vi "User events.vi"() -> (0 "error out":errorcluster, 3 "User events":T1)   [LabVIEW 2020, in "Arduino stepper.lvlib"]
uses:
  Arduino stepper.lvlib
  Wake HL args--typedef.ctl
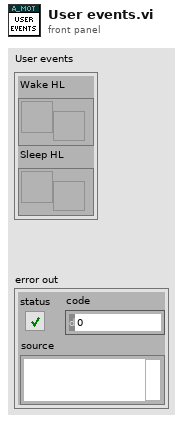
[diagram p1: front panel]
types:
  T1 = cluster{"Wake HL":refnum<user-event>, "Sleep HL":refnum<user-event>}
  T2 = typedef "Arduino stepper.lvlib/Wake HL args--typedef.ctl" = cluster{"VISA resource name":refnum<visa-resource-name>, "Timeout":i32, "Module ID":i32}
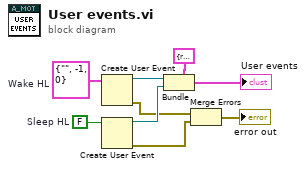
[diagram p0: block diagram]
diagram:
  w6 = T2 {"VISA resource name"="", "Timeout"=-1, "Module ID"=0}  # Wake HL
  w7 = FALSE  # Sleep HL
  n1 = Create User Event(user event datatype=w6) -> (user event=w8:refnum<user-event>, error out=w5:errorcluster)  [unwired: 1 in]
  n2 = Create User Event(user event datatype=w7) -> (user event=w9:refnum<user-event>, error out=w4:errorcluster)  [unwired: 1 in]
  n3 = Bundle(cluster=T1 {"Wake HL"=refnum, "Sleep HL"=refnum} ("output cluster"), "Wake HL"=w8, "Sleep HL"=w9) -> (→"User events":T1)
  n4 = Merge Errors(w5, w4) -> (→"error out":errorcluster)
